vi "Test Get In User Documents.vi"() -> ()   [LabVIEW 2021, in "Path Utilities.lvlib"]
doc: "Unit Test for \"Get In User Documents.vi\"."
uses:
  Path Utilities.lvlib
panel:
  in  "User Name":string="Thomas"
  out "error out":errorcluster
  out "Pass - System Path with Base":bool
  out "Result - System Path with Base":path
  out "Expected - System Path with Base":path
  out "Pass - System Path Only":bool
  out "Result - System Path Only":path
  out "Expected - System Path Only":path
  in  "Base Path":path=path "Company/Application"
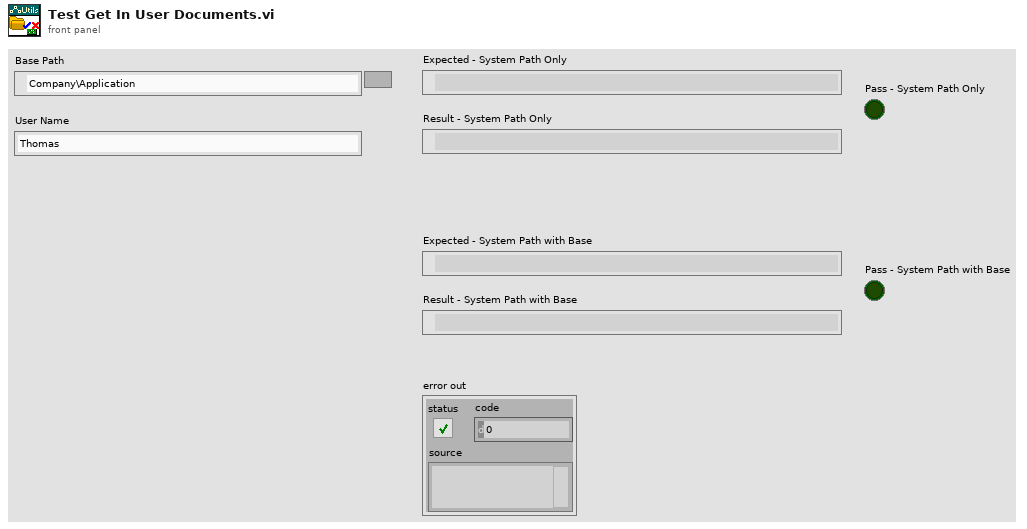
[diagram p1: front panel]
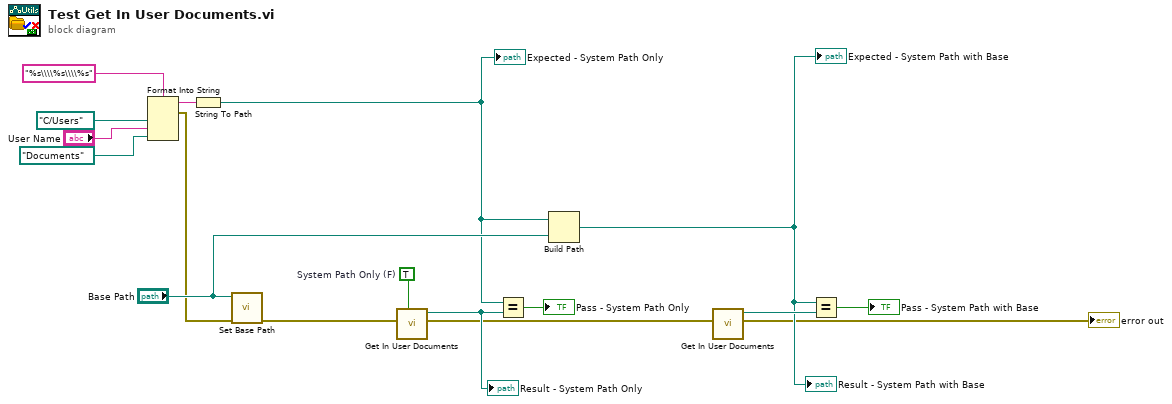
[diagram p0: block diagram]
diagram:
  w16 = TRUE  # System Path Only (F)
  n1 = Format Into String(format string="%s\\\\%s\\\\%s", path "C:/Users", "User Name", path "Documents") -> (resulting string=w4:string, error out=w2:errorcluster)  [unwired: 2 in]
  n2 = String To Path(string=w4) -> (path=w1:path)
  "Expected - System Path Only" <- w1
  n3 = call "Set Base Path.vi"("error in (no error)"=w2, "Base Path"="Base Path") -> ("error out"=w17:errorcluster)  [unwired: 8 in, 1 out]
  n4 = call "Get In User Documents.vi"("System Path Only (F)"=w16, "error in (no error)"=w17) -> ("error out"=w13:errorcluster, "Path"=w14:path)  [unwired: 8 in]
  "Result - System Path Only" <- w14
  n5 = Equal?(x=w1, y=w14) -> (x = y?=→"Pass - System Path Only":bool)
  n6 = Build Path(base path=w1, name or relative path="Base Path") -> (appended path=w9:path)
  "Expected - System Path with Base" <- w9
  "Result - System Path with Base" <- w9
  n7 = call "Get In User Documents.vi"("error in (no error)"=w13) -> ("error out"=→"error out":errorcluster, "Path"=w11:path)  [unwired: 9 in]
  n8 = Equal?(x=w9, y=w11) -> (x = y?=→"Pass - System Path with Base":bool)
